vi "Build Command.vi"(10 "Command Definition":T1) -> (2 "Command":string)   [LabVIEW 2018, in "Collaborator.lvlib"]
uses:
  Collaborator.lvlib
  Command Configuration.ctl
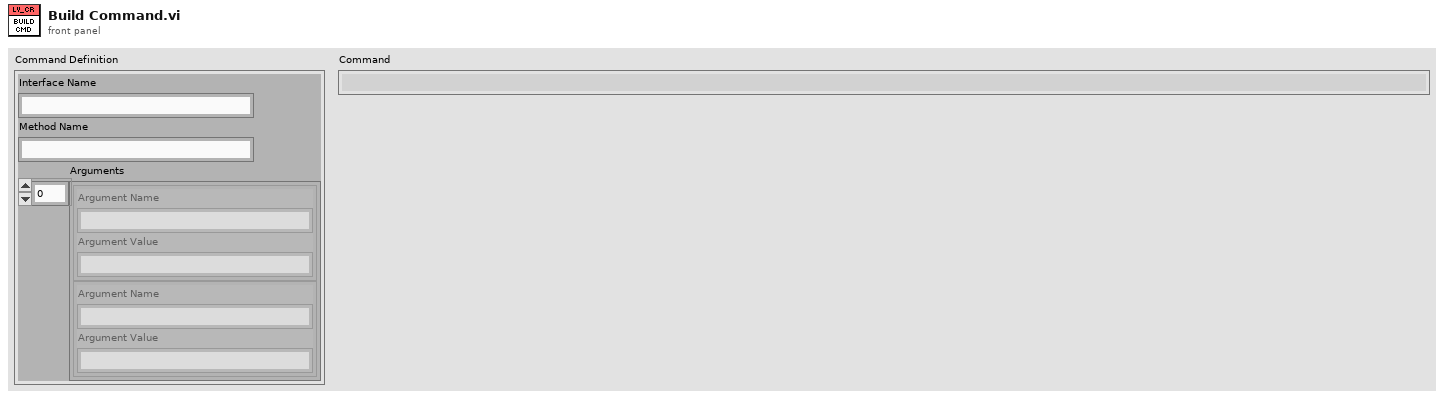
[diagram p1: front panel]
types:
  T1 = typedef "Command Configuration.ctl" = cluster{"Interface Name":string, "Method Name":string, "Arguments":cluster{"Argument Name":string, "Argument Value":string}[]}
  T2 = cluster{"Argument Name":string, "Argument Value":string}[]
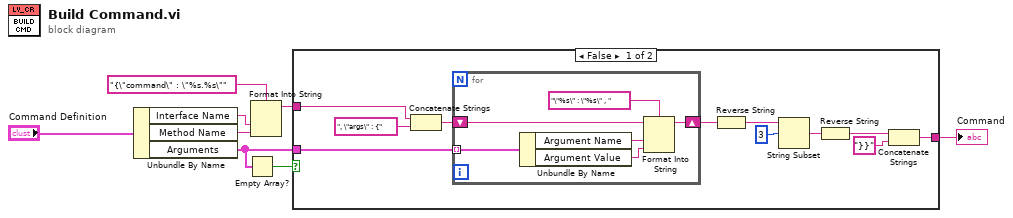
[diagram p0: block diagram]
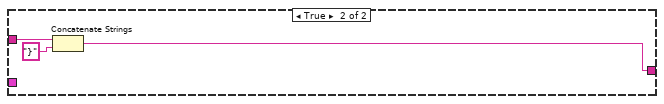
[diagram p2: hidden frame]
diagram:
  n1 = Unbundle By Name("Command Definition") -> ("Interface Name"=w6:string, "Method Name"=w5:string, "Arguments"=w2:T2)
  n2 = Empty Array?(array=w2) -> (empty?=w4:bool)
  n3 = Format Into String(format string="{\"command\" : \"%s.%s\"", w6, w5) -> (resulting string=w3:string)  [unwired: 2 in, 1 out]
  n4 = case shown="False" w4 {
    tunnel: w3 -> [w19 w28]
    tunnel: [w9 w26] -> w1
    tunnel: w2 -> [w16 _]
    frame False {
      n5 = Concatenate Strings(w19, ", \"args\" : {" ("format string")) -> (w17:string)
      n6 = for {
        shift-right: [w20] -> w15
        shift-left: w17 -> [w22]
        tunnel: w16 -> [w25] mode=indexing
        n7 = Unbundle By Name(w25) -> ("Argument Name"=w24:string, "Argument Value"=w23:string)
        n8 = Format Into String(format string="\"%s\" : \"%s\" , ", initial string=w22, w24, w23) -> (resulting string=w20:string)  [unwired: 1 in, 1 out]
      }
      n9 = Reverse String(1:w15) -> (0:w14:string)
      n10 = String Subset(string=w14, offset (0)=3) -> (substring=w12:string)  [unwired: 1 in]
      n11 = Reverse String(1:w12) -> (0:w11:string)
      n12 = Concatenate Strings(w11, "}}" ("string")) -> (w9:string)
    }
    frame True {
      n13 = Concatenate Strings(w28, "}" ("string")) -> (w26:string)
    }
  }
  "Command" <- w1
